vi "Convert String To Digital.vi"(8 "error in (no error)":errorcluster, 10 "Value":string, 11 "DigNum Refnum":refnum<vi>) -> (0 "error out":errorcluster)   [LabVIEW 2021, in "CANOpen Addon System Explorer.lvlib"]
uses:
  CANOpen Addon System Explorer.lvlib
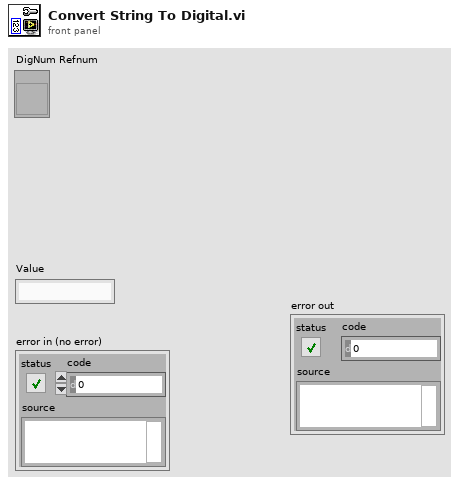
[diagram p1: front panel]
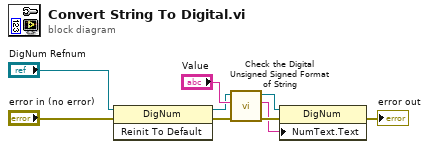
[diagram p0: block diagram]
diagram:
  n1 = invoke class="DigNum" method="Reinit To Default"(reference="DigNum Refnum", error in="error in (no error)") -> (reference out=w4:refnum<vi>, error out=w6:errorcluster)  [unwired: 1 in, 1 out]
  n2 = call "Check the Digital Unsigned Signed Format of String.vi"("error in (no error)"=w6, "Value"="Value", "DigNum Refnum"=w4) -> ("error out"=w5:errorcluster, "Valuse Without Flag"=w2:string, "dup DigNum Refnum"=w3:refnum<vi>)  [unwired: 6 in]
  n3 = property class="DigNum"(reference=w3, error in=w5, "NumText.Text"=w2) -> (error out=→"error out":errorcluster)  [unwired: 1 out]
